vi "Destroy REST Client.vi"(8 "error in (no error)":errorcluster, 11 "REST Client in":refnum<class "REST Client.lvclass">) -> (0 "error out":errorcluster)   [LabVIEW 2020, in "REST Client.lvlib" / "REST Client.lvclass"]
doc: "Destroy REST client reference."
uses:
  REST Client.lvclass
  REST Client.lvclass/REST Client.ctl
  <vilib>/VIPM Community/HTTP Client Plugin - Base/Classes/Abstract HTTP Client/Abstract HTTP Client.lvclass
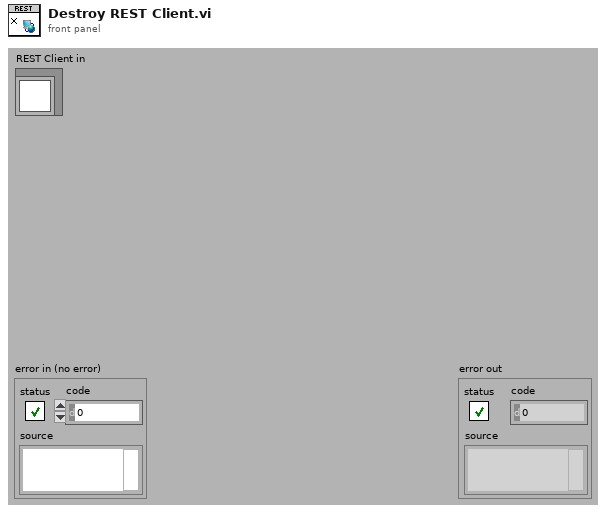
[diagram p1: front panel]
types:
  T1 = typedef "REST Client.lvlib/REST Client.lvclass/HTTP Header.ctl" = cluster{"header":T2, "value":string}
  T2 = typedef "lib_NI_Advanced HTTP Client.lvlib/Session.lvclass/Header--Combo Box.ctl" = string
  T3 = cluster{"HTTP Client Abstract.lvlib:Abstract HTTP Client.lvclass":refnum<class "Abstract HTTP Client.lvclass">, "Default Headers ([JSON])":T1[]}[]
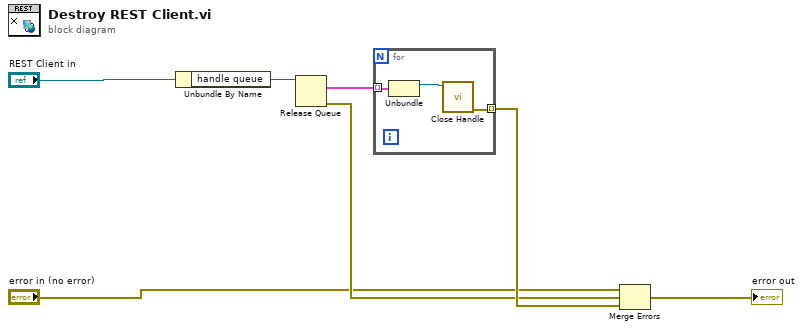
[diagram p0: block diagram]
diagram:
  n1 = Unbundle By Name("REST Client in") -> ("handle queue"=w6:refnum<queue>)
  n2 = Release Queue(queue=w6) -> (remaining elements=w5:T3, error out=w2:errorcluster)  [unwired: 2 in, 1 out]
  n3 = for {
    tunnel: w5 -> [w10] mode=indexing
    tunnel: [w8] -> w3 mode=indexing
    n4 = Unbundle(w10) -> ("HTTP Client Abstract.lvlib:Abstract HTTP Client.lvclass"=w9:refnum<class "Abstract HTTP Client.lvclass">)  [unwired: 1 out]
    n5 = call-dynamic "Close Handle.vi"("HTTP Client Abstract in"=w9) -> ("error out"=w8:errorcluster)  [unwired: 9 in, 1 out]
  }
  n6 = Merge Errors("error in (no error)", w2, w3) -> (→"error out":errorcluster)
